vi "最終版.vi"() -> ()   [LabVIEW 2014]
uses:
  cloud.ctl
  heart.ctl
  <vilib>/Utility/inputDevices.llb/keyboardAcquire.vi
  <vilib>/Utility/inputDevices.llb/closeKeyboard.vi
panel:
  out "2-2":T1
  out "2-1":T2
  out "2":T1
  out "1":T2
  out "User 1":T3
  out "User 2":T3
  out "Ring 6":T4
  out "Ring 5":T5
  out "Ring 4":T5
  out "Ring 3":T4
  out "2jump":bool=TRUE
  out "User2 name":string
  out "User1 name":string
  out "人1生命":dbl
  out "人2生命":dbl
  out "heart 6":T6
  out "heart 5":T6
  out "heart 4":T6
  out "heart 3":T6
  out "heart 2":T6
  out "heart 1":T6
  out "雲  3":T7
  out "black hole":T8
  out "雲 2":T7
  out "雲":T7
  out "1jump":bool=TRUE
  out "火右飛 2":bool=TRUE
  out "火左飛 2":bool
  out "火左飛":bool
  out "火右飛":bool=TRUE
  in  "stop jump2":bool
  in  "stop jump1":bool
  in  "right/left 2":bool
  in  "人2":bool
  in  "right/left":bool
  in  "人1":bool
  in  "整個遊戲中止":bool
  # "587"
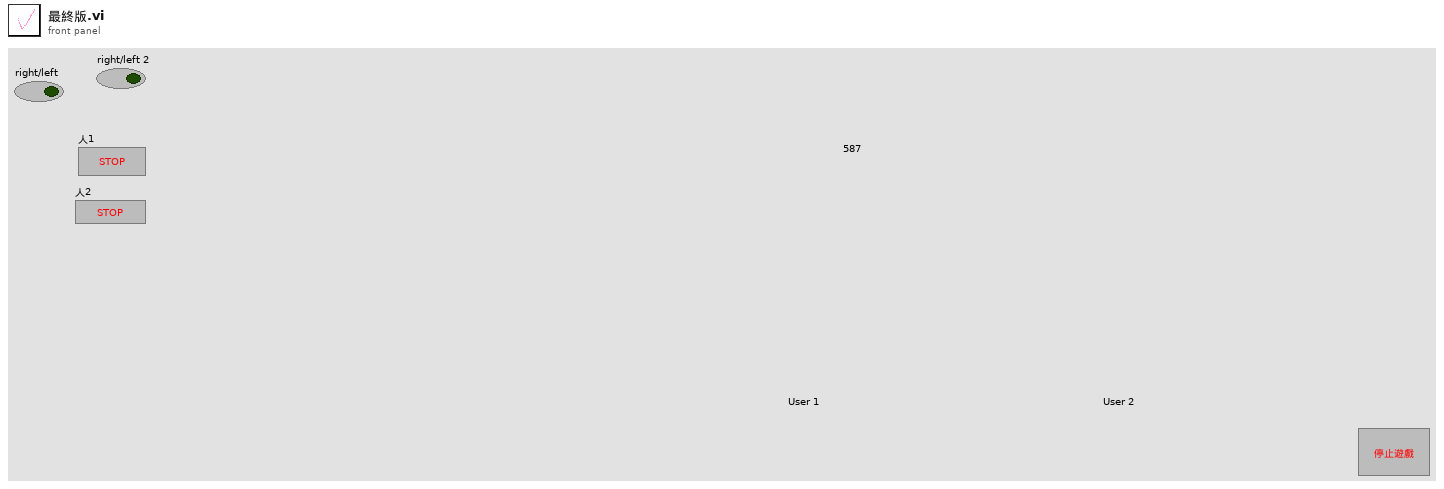
[diagram p1: front panel]
types:
  T1 = typedef "火焰2.ctl" = u16
  T2 = typedef "火焰.ctl" = u16
  T3 = typedef "Control 3.ctl" = u16
  T4 = typedef "窄短cloud.ctl" = u16
  T5 = typedef "窄cloud.ctl" = u16
  T6 = typedef "heart.ctl" = u16
  T7 = typedef "cloud.ctl" = u16
  T8 = typedef "Control 4.ctl" = u16
  T9 = enum16{"0", "1", "2", "3", "4", "5", "6", "7", "8", "9", "A", "B", "C", "D", "E", "F", "G", "H", "I", "J", "K", "L", "M", "N", "O", "P", "Q", "R", "S", "T", "U", "V", "W", "X", "Y", "Z", "F1", "F2", "F3", "F4", "F5", "F6", "F7", "F8", "F9", "F10", "F11", "F12", "F13", "F14", "F15", "ADD", "BACK", "BACKSLASH", "CAPITAL", "COMMA", "DECIMAL", "DELETE", "DIVIDE", "DOWN", "END", "EQUALS", "ESCAPE", "GRAVE (`)", "HOME", "INSERT", "LBRACKET", "LCONTROL", "LEFT", "L ALT", "LSHIFT", "LWIN", "MINUS", "MULTIPLY", "NEXT", "NUMLOCK", "NUMPAD_0", "NUMPAD_1", "NUMPAD_2", "NUMPAD_3", "NUMPAD_4", "NUMPAD_5", "NUMPAD_6", "NUMPAD_7", "NUMPAD_8", "NUMPAD_9", "PAUSE", "PERIOD", "PRIOR (PG UP)", "RBRACKET", "RCONTROL", "RETURN", "RIGHT", "R ALT", "RSHIFT", "RWIN", "SCROLL", "SEMICOLON", "SLASH", "SPACE", "SUBTRACT", "TAB", "UP", "ENTER (num pad)", "' (quote)"}
  T10 = enum16{"0", "1", "2", "3", "4", "5", "6", "7", "8", "9", "A", "B", "C", "D", "E", "F", "G", "H", "I", "J", "K", "L", "M", "N", "O", "P", "Q", "R", "S", "T", "U", "V", "W", "X", "Y", "Z", "F1", "F2", "F3", "F4", "F5", "F6", "F7", "F8", "F9", "F10", "F11", "F12", "F13", "F14", "F15", "ADD", "BACK", "BACKSLASH", "CAPITAL", "COMMA", "DECIMAL", "DELETE", "DIVIDE", "DOWN", "END", "EQUALS", "ESCAPE", "GRAVE (`)", "HOME", "INSERT", "LBRACKET", "LCONTROL", "LEFT", "L ALT", "LSHIFT", "LWIN", "MINUS", "MULTIPLY", "NEXT", "NUMLOCK", "NUMPAD_0", "NUMPAD_1", "NUMPAD_2", "NUMPAD_3", "NUMPAD_4", "NUMPAD_5", "NUMPAD_6", "NUMPAD_7", "NUMPAD_8", "NUMPAD_9", "PAUSE", "PERIOD", "PRIOR (PG UP)", "RBRACKET", "RCONTROL", "RETURN", "RIGHT", "R ALT", "RSHIFT", "RWIN", "SCROLL", "SEMICOLON", "SLASH", "SPACE", "SUBTRACT", "TAB", "UP", "ENTER (num pad)", "' (quote)"}[]
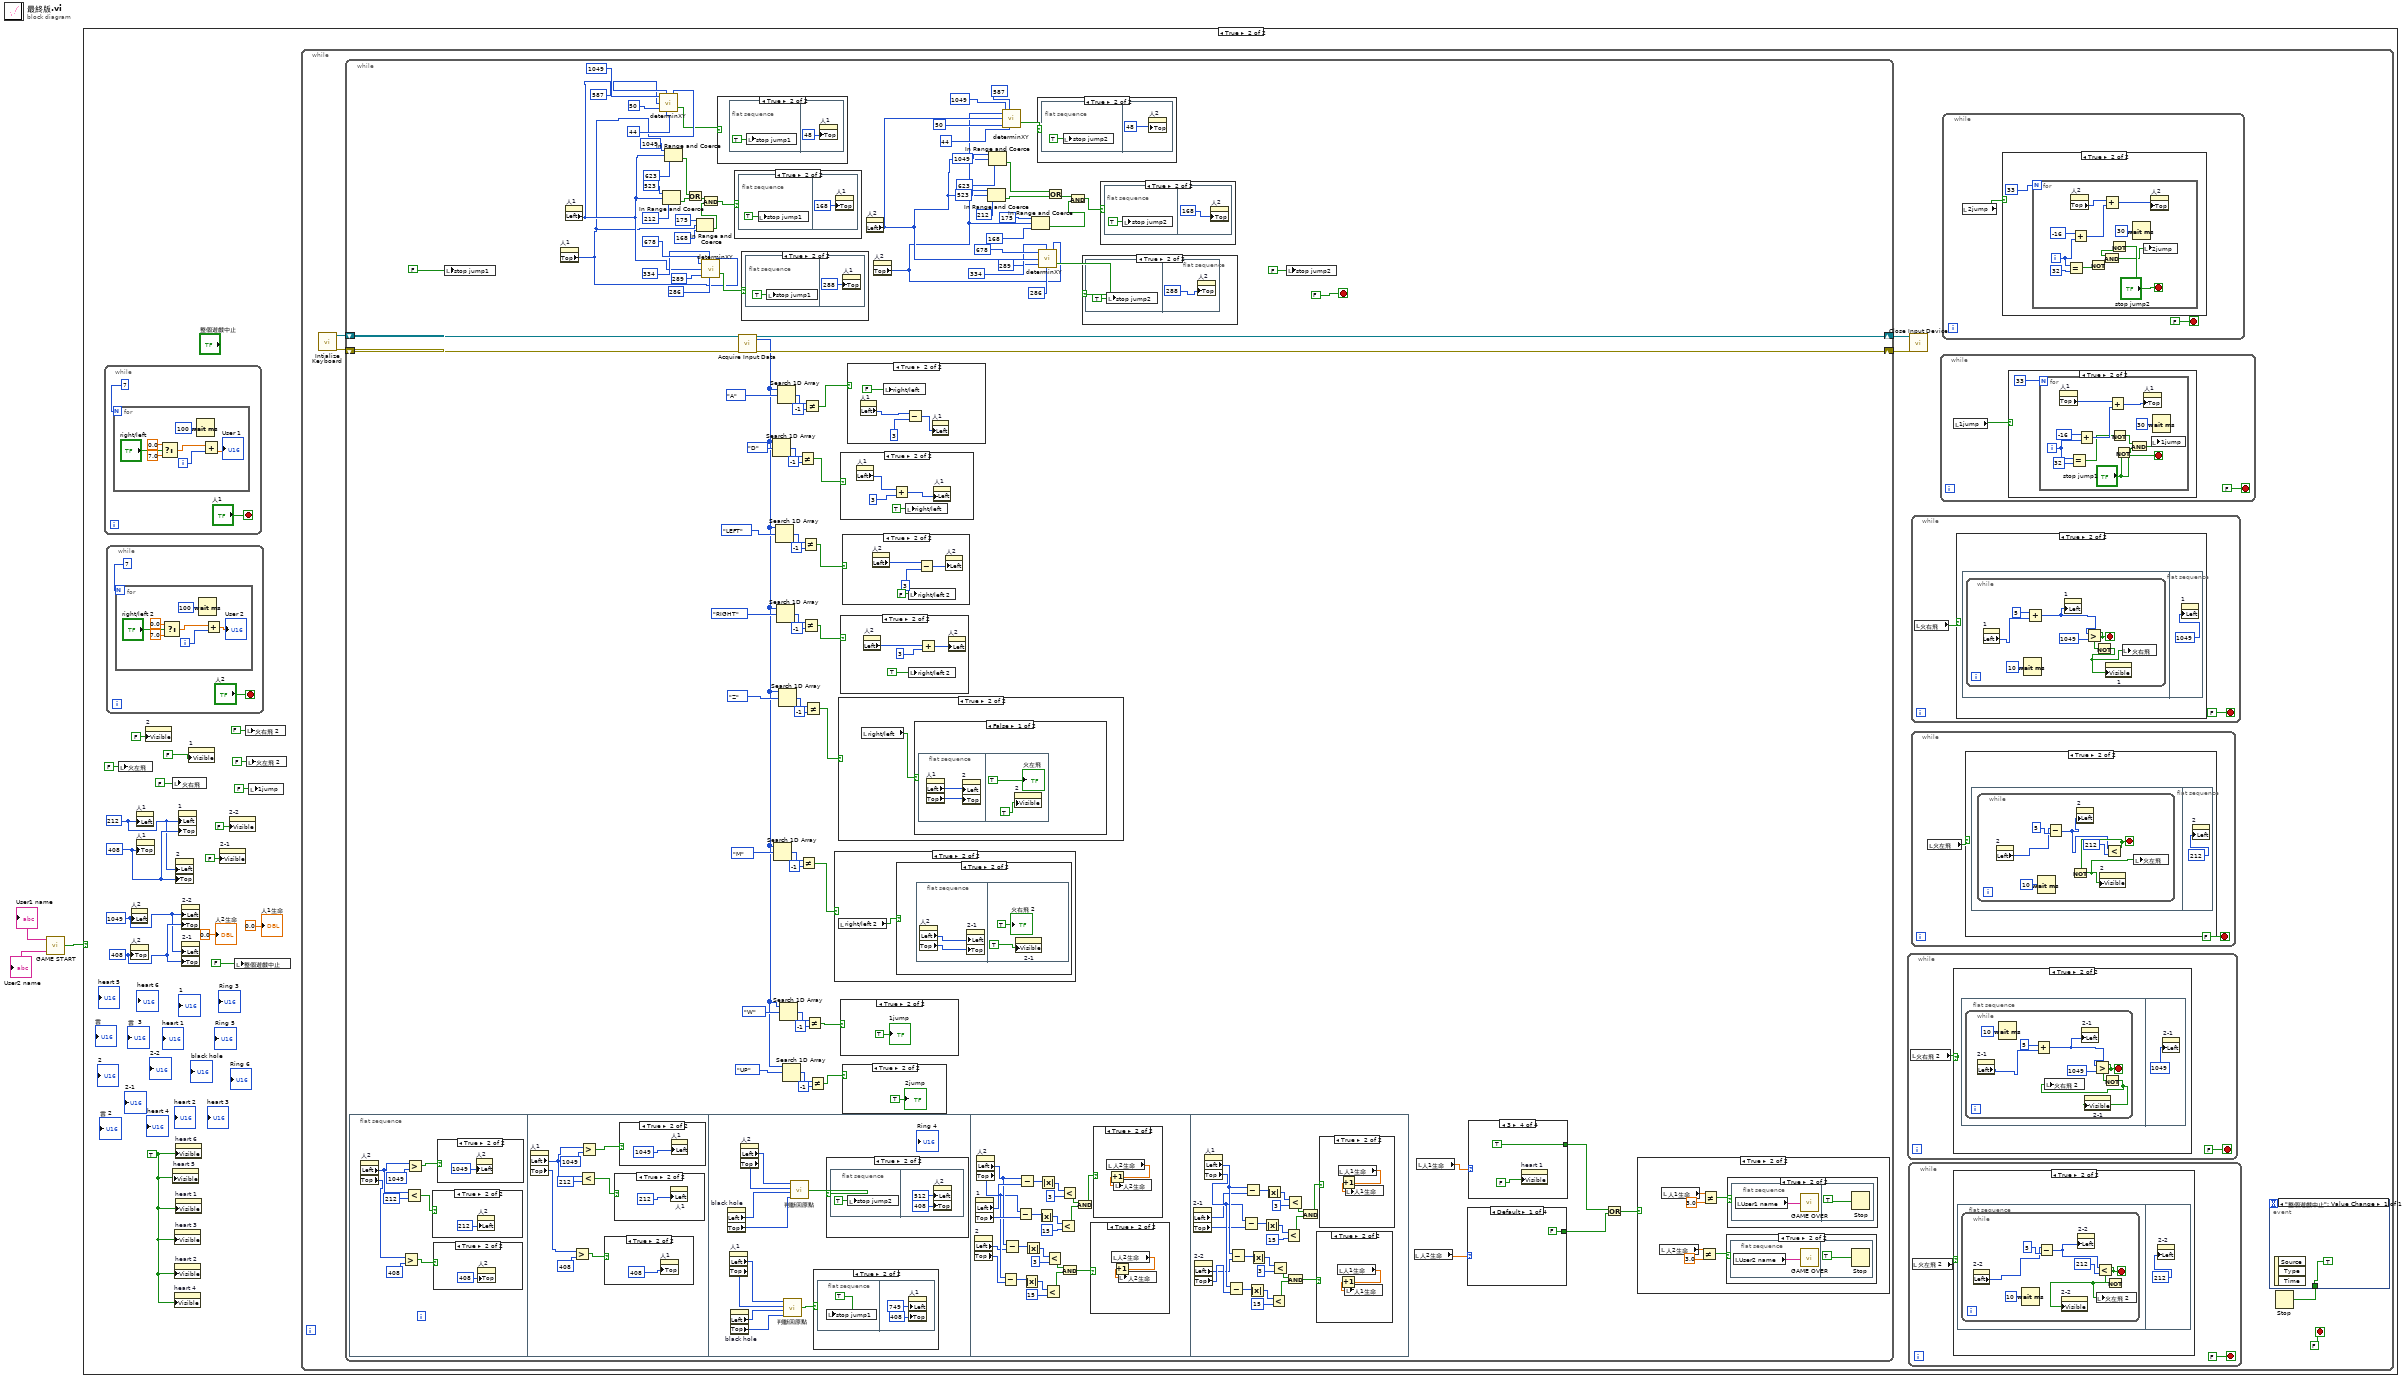
[diagram p0: block diagram]
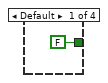
[diagram p13: hidden frame]
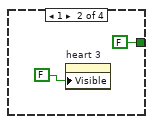
[diagram p14: hidden frame]
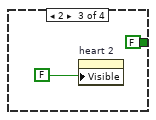
[diagram p15: hidden frame]
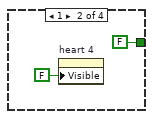
[diagram p16: hidden frame]
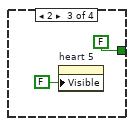
[diagram p17: hidden frame]
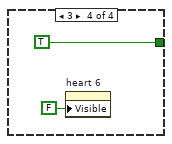
[diagram p18: hidden frame]
diagram:
  n1 = call "GAME START.vi"() -> ("stop 2"=w3:bool, "User2 name 2"=→"User2 name":string, "User1 name 2"=→"User1 name":string)  [unwired: 1 in]
  n2 = case shown="True" w3 {
    frame False {
    }
    frame True {
      w4 = TRUE ("Visible")
      w15 = 408 ("Position:Top")
      w14 = 1049 ("Position:Left")
      w13 = 408 ("Position:Top")
      w12 = 212 ("Position:Left")
      n3 = while {
        stop <- "人1" stop-if-true
        n4 = for {
          N: 7 -> [_]
          i -> [w28]
          n5 = Select(t=0.0, s="right/left", f=7.0) -> (s? t:f=w25:dbl)
          n6 = Wait (ms)(milliseconds to wait=u32 100) -> ()  [unwired: 1 out]
          n7 = Add(x=w25, y=w28) -> (x+y=→"User 1":dbl)
        }
      }
      n8 = while {
        stop <- "人2" stop-if-true
        n9 = for {
          N: 7 -> [_]
          i -> [w37]
          n10 = Select(t=0.0, s="right/left 2", f=7.0) -> (s? t:f=w35:dbl)
          n11 = Wait (ms)(milliseconds to wait=u32 100) -> ()  [unwired: 1 out]
          n12 = Add(x=w35, y=w37) -> (x+y=→"User 2":dbl)
        }
      }
      n13 = local write "火左飛"(FALSE ("火左飛")) -> ()
      n14 = property on="人2" class="Ring (strict)"("Top"=w15) -> ()  [unwired: 2 in, 2 out]
      n15 = property on="人2" class="Ring (strict)"("Left"=w14) -> ()  [unwired: 2 in, 2 out]
      n16 = property on="人1" class="Ring (strict)"("Left"=w12) -> ()  [unwired: 2 in, 2 out]
      n17 = property on="人1" class="Ring (strict)"("Top"=w13) -> ()  [unwired: 2 in, 2 out]
      n18 = property on="2" class="Ring (strict)"("Visible"=FALSE) -> ()  [unwired: 2 in, 2 out]
      n19 = local write "火右飛"(FALSE ("Boolean")) -> ()
      n20 = property on="heart 5" class="Ring (strict)"("Visible"=w4) -> ()  [unwired: 2 in, 2 out]
      n21 = property on="heart 4" class="Ring (strict)"("Visible"=w4) -> ()  [unwired: 2 in, 2 out]
      n22 = property on="heart 3" class="Ring (strict)"("Visible"=w4) -> ()  [unwired: 2 in, 2 out]
      n23 = property on="heart 2" class="Ring (strict)"("Visible"=w4) -> ()  [unwired: 2 in, 2 out]
      n24 = property on="heart 6" class="Ring (strict)"("Visible"=w4) -> ()  [unwired: 2 in, 2 out]
      n25 = property on="heart 1" class="Ring (strict)"("Visible"=w4) -> ()  [unwired: 2 in, 2 out]
      n26 = property on="2" class="Ring (strict)"("Left"=w12, "Top"=w13) -> ()  [unwired: 2 in, 2 out]
      n27 = property on="1" class="Ring (strict)"("Left"=w12, "Top"=w13) -> ()  [unwired: 2 in, 2 out]
      n28 = property on="2-2" class="Ring (strict)"("Left"=w14, "Top"=w15) -> ()  [unwired: 2 in, 2 out]
      n29 = property on="2-1" class="Ring (strict)"("Left"=w14, "Top"=w15) -> ()  [unwired: 2 in, 2 out]
      n30 = property on="1" class="Ring (strict)"("Visible"=FALSE) -> ()  [unwired: 2 in, 2 out]
      n31 = property on="2-1" class="Ring (strict)"("Visible"=FALSE) -> ()  [unwired: 2 in, 2 out]
      n32 = property on="2-2" class="Ring (strict)"("Visible"=FALSE) -> ()  [unwired: 2 in, 2 out]
      n33 = local write "整個遊戲中止"(FALSE ("整個遊戲中止")) -> ()
      n34 = local write "火右飛 2"(FALSE ("火右飛 2")) -> ()
      n35 = local write "火左飛 2"(FALSE ("火左飛 2")) -> ()
      n36 = local write "1jump"(FALSE ("1jump")) -> ()
      n37 = while {
        stop <- FALSE stop-if-true
        n38 = call <vilib>:"Intialize Keyboard.vi"() -> ("error out"=w43:errorcluster, "device ID"=w44:refnum<k1>)  [unwired: 10 in]
        n39 = while {
          shift-right: [w206] -> w41
          shift-left: w44 -> [w203]
          shift-right: [w205] -> w42
          shift-left: w43 -> [w204]
          stop <- FALSE stop-if-true
          n40 = flat-sequence {
            frame #0 {
              n41 = property on="人2" class="Ring (strict)"() -> ("Left"=w238:i32, "Top"=w233:i32)  [unwired: 2 in, 2 out]
              n42 = Greater?(x=w233, y=408) -> (0:w232:bool)
              n43 = Less?(x=w238, y=212) -> (x < y?=w235:bool)
              n44 = Greater?(x=w238, y=1049) -> (0:w236:bool)
              n45 = case shown="True" w235 {
                frame False {
                }
                frame True {
                  n46 = property on="人2" class="Ring (strict)"("Left"=212 ("Position:Left")) -> ()  [unwired: 2 in, 2 out]
                }
              }
              n47 = case shown="True" w232 {
                frame False {
                }
                frame True {
                  n48 = property on="人2" class="Ring (strict)"("Top"=408 ("Position:Left")) -> ()  [unwired: 2 in, 2 out]
                }
              }
              n49 = case shown="True" w236 {
                frame False {
                }
                frame True {
                  n50 = property on="人2" class="Ring (strict)"("Left"=1049 ("Position:Left")) -> ()  [unwired: 2 in, 2 out]
                }
              }
            }
            frame #1 {
              n51 = property on="人1" class="Ring (strict)"() -> ("Left"=w250:i32, "Top"=w243:i32)  [unwired: 2 in, 2 out]
              n52 = Greater?(x=w243, y=408) -> (0:w245:bool)
              n53 = Less?(x=w250, y=212) -> (x < y?=w249:bool)
              n54 = Greater?(x=w250, y=1049) -> (0:w248:bool)
              n55 = case shown="True" w245 {
                frame False {
                }
                frame True {
                  n56 = property on="人1" class="Ring (strict)"("Top"=408 ("Position:Left")) -> ()  [unwired: 2 in, 2 out]
                }
              }
              n57 = case shown="True" w249 {
                frame False {
                }
                frame True {
                  n58 = property on="人1" class="Ring (strict)"("Left"=212 ("Position:Left")) -> ()  [unwired: 2 in, 2 out]
                }
              }
              n59 = case shown="True" w248 {
                frame False {
                }
                frame True {
                  n60 = property on="人1" class="Ring (strict)"("Left"=1049 ("Position:Left")) -> ()  [unwired: 2 in, 2 out]
                }
              }
            }
            frame #2 {
              n61 = property on="black hole" class="Ring (strict)"() -> ("Left"=w261:i32, "Top"=w260:i32)  [unwired: 2 in, 2 out]
              n62 = property on="人1" class="Ring (strict)"() -> ("Left"=w254:i32, "Top"=w255:i32)  [unwired: 2 in, 2 out]
              n63 = property on="black hole" class="Ring (strict)"() -> ("Left"=w256:i32, "Top"=w257:i32)  [unwired: 2 in, 2 out]
              n64 = property on="人2" class="Ring (strict)"() -> ("Left"=w263:i32, "Top"=w262:i32)  [unwired: 2 in, 2 out]
              n65 = call "判斷回原點.vi"("¬}y"=w257, "¬}x"=w256, "人y"=w255, "人x"=w254) -> ("x .and. y?"=w258:bool)
              n66 = call "判斷回原點.vi"("¬}y"=w260, "¬}x"=w261, "人y"=w262, "人x"=w263) -> ("x .and. y?"=w259:bool)
              n67 = case shown="True" w258 {
                frame False {
                }
                frame True {
                  n68 = flat-sequence {
                    frame #0 {
                      n69 = local write "stop jump1"(TRUE) -> ()
                    }
                    frame #1 {
                      n70 = property on="人1" class="Ring (strict)"("Left"=749 ("Position:Left"), "Top"=408 ("Position:Top")) -> ()  [unwired: 2 in, 2 out]
                    }
                  }
                }
              }
              n71 = case shown="True" w259 {
                frame False {
                }
                frame True {
                  n72 = flat-sequence {
                    frame #0 {
                      n73 = local write "stop jump2"(TRUE ("stop jump2")) -> ()
                    }
                    frame #1 {
                      n74 = property on="人2" class="Ring (strict)"("Left"=512 ("Position:Left"), "Top"=408 ("Position:Top")) -> ()  [unwired: 2 in, 2 out]
                    }
                  }
                }
              }
            }
            frame #3 {
              n75 = property on="2" class="Ring (strict)"() -> ("Left"=w271:i32, "Top"=w270:i32)  [unwired: 2 in, 2 out]
              n76 = property on="1" class="Ring (strict)"() -> ("Left"=w293:i32, "Top"=w286:i32)  [unwired: 2 in, 2 out]
              n77 = property on="人2" class="Ring (strict)"() -> ("Left"=w273:i32, "Top"=w272:i32)  [unwired: 2 in, 2 out]
              n78 = Subtract(x=w272, y=w270) -> (x-y=w280:i32)
              n79 = Subtract(x=w273, y=w271) -> (x-y=w275:i32)
              n80 = Subtract(x=w272, y=w286) -> (x-y=w287:i32)
              n81 = Subtract(x=w273, y=w293) -> (x-y=w292:i32)
              n82 = Absolute Value(x=w280) -> (abs(x)=w279:i32)
              n83 = Absolute Value(x=w275) -> (abs(x)=w276:i32)
              n84 = Absolute Value(x=w287) -> (abs(x)=w288:i32)
              n85 = Absolute Value(x=w292) -> (abs(x)=w291:i32)
              n86 = Less?(x=w279, y=15) -> (x < y?=w282:bool)
              n87 = Less?(x=w276, y=3) -> (x < y?=w281:bool)
              n88 = Less?(x=w288, y=15) -> (x < y?=w284:bool)
              n89 = Less?(x=w291, y=3) -> (x < y?=w285:bool)
              n90 = And(x=w281, y=w282) -> (x .and. y?=w274:bool)
              n91 = And(x=w285, y=w284) -> (x .and. y?=w283:bool)
              n92 = case shown="True" w274 {
                frame False {
                }
                frame True {
                  n93 = local read "人2生命"() -> (w295:dbl)
                  n94 = Increment(x=w295) -> (x+1=w294:dbl)
                  n95 = local write "人2生命"(w294) -> ()
                }
              }
              n96 = case shown="True" w283 {
                frame False {
                }
                frame True {
                  n97 = local read "人2生命"() -> (w296:dbl)
                  n98 = Increment(x=w296) -> (x+1=w297:dbl)
                  n99 = local write "人2生命"(w297) -> ()
                }
              }
            }
            frame #4 {
              n100 = property on="2-1" class="Ring (strict)"() -> ("Left"=w300:i32, "Top"=w301:i32)  [unwired: 2 in, 2 out]
              n101 = property on="2-2" class="Ring (strict)"() -> ("Left"=w298:i32, "Top"=w299:i32)  [unwired: 2 in, 2 out]
              n102 = property on="人1" class="Ring (strict)"() -> ("Left"=w303:i32, "Top"=w302:i32)  [unwired: 2 in, 2 out]
              n103 = Subtract(x=w302, y=w299) -> (x-y=w315:i32)
              n104 = Subtract(x=w303, y=w298) -> (x-y=w320:i32)
              n105 = Subtract(x=w302, y=w301) -> (x-y=w309:i32)
              n106 = Subtract(x=w303, y=w300) -> (x-y=w304:i32)
              n107 = Absolute Value(x=w315) -> (abs(x)=w316:i32)
              n108 = Absolute Value(x=w320) -> (abs(x)=w319:i32)
              n109 = Absolute Value(x=w309) -> (abs(x)=w308:i32)
              n110 = Absolute Value(x=w304) -> (abs(x)=w305:i32)
              n111 = Less?(x=w316, y=15) -> (x < y?=w313:bool)
              n112 = Less?(x=w319, y=3) -> (x < y?=w314:bool)
              n113 = Less?(x=w308, y=15) -> (x < y?=w311:bool)
              n114 = Less?(x=w305, y=3) -> (x < y?=w310:bool)
              n115 = And(x=w314, y=w313) -> (x .and. y?=w321:bool)
              n116 = And(x=w310, y=w311) -> (x .and. y?=w312:bool)
              n117 = case shown="True" w321 {
                frame False {
                }
                frame True {
                  n118 = local read "人1生命"() -> (w323:dbl)
                  n119 = Increment(x=w323) -> (x+1=w322:dbl)
                  n120 = local write "人1生命"(w322) -> ()
                }
              }
              n121 = case shown="True" w312 {
                frame False {
                }
                frame True {
                  n122 = local read "人1生命"() -> (w324:dbl)
                  n123 = Increment(x=w324) -> (x+1=w325:dbl)
                  n124 = local write "人1生命"(w325) -> ()
                }
              }
            }
          }
          n125 = local write "stop jump1"(FALSE ("stop jump1")) -> ()
          n126 = property on="人1" class="Ring (strict)"() -> ("Top"=w139:i32)  [unwired: 2 in, 2 out]
          n127 = property on="人1" class="Ring (strict)"() -> ("Left"=w142:i32)  [unwired: 2 in, 2 out]
          n128 = call "determinXY.vi"("x max"=1049 ("upper limit"), "x min"=587 ("lower limit"), "x"=w142, "y max"=50 ("upper limit"), "y min"=44 ("lower limit"), "y"=w139) -> ("result"=w138:bool)
          n129 = In Range and Coerce(upper limit=523, x=w142, lower limit=212) -> (In Range?=w177:bool)  [unwired: 1 out]
          n130 = In Range and Coerce(upper limit=1049, x=w142, lower limit=623) -> (In Range?=w178:bool)  [unwired: 1 out]
          n131 = Or(x=w178, y=w177) -> (x .or. y?=w179:bool)
          n132 = In Range and Coerce(upper limit=175, x=w139, lower limit=168 ("y")) -> (In Range?=w183:bool)  [unwired: 1 out]
          n133 = And(x=w179, y=w183) -> (x .and. y?=w176:bool)
          n134 = call "determinXY.vi"("x max"=678 ("upper limit"), "x min"=334 ("lower limit"), "x"=w142, "y max"=289 ("upper limit"), "y min"=286 ("y"), "y"=w139) -> ("result"=w145:bool)
          n135 = case shown="True" w138 {
            frame False {
            }
            frame True {
              n136 = flat-sequence {
                frame #0 {
                  n137 = local write "stop jump1"(TRUE ("stop jump1")) -> ()
                }
                frame #1 {
                  n138 = property on="人1" class="Ring (strict)"("Top"=48 ("Position:Top")) -> ()  [unwired: 2 in, 2 out]
                }
              }
            }
          }
          n139 = case shown="True" w176 {
            frame False {
            }
            frame True {
              n140 = flat-sequence {
                frame #0 {
                  n141 = local write "stop jump1"(TRUE ("stop jump1")) -> ()
                }
                frame #1 {
                  n142 = property on="人1" class="Ring (strict)"("Top"=168 ("Position:Top")) -> ()  [unwired: 2 in, 2 out]
                }
              }
            }
          }
          n143 = call-poly <vilib>:"Acquire Input Data.vi"("device ID"=w203, "error in (no error)"=w204) -> ("device ID"=w206:refnum<k1>, "keys pressed"=w119:T10, "error out"=w205:errorcluster)  [unwired: 15 in]
          n144 = case shown="True" w145 {
            frame False {
            }
            frame True {
              n145 = flat-sequence {
                frame #0 {
                  n146 = local write "stop jump1"(TRUE ("stop jump1")) -> ()
                }
                frame #1 {
                  n147 = property on="人1" class="Ring (strict)"("Top"=288 ("Position:Top")) -> ()  [unwired: 2 in, 2 out]
                }
              }
            }
          }
          n148 = Search 1D Array(1D array=w119, element=T9."D") -> (index of element=w197:i32)  [unwired: 1 in]
          n149 = Search 1D Array(1D array=w119, element=T9."M") -> (index of element=w159:i32)  [unwired: 1 in]
          n150 = Search 1D Array(1D array=w119, element=T9."LEFT") -> (index of element=w194:i32)  [unwired: 1 in]
          n151 = Search 1D Array(1D array=w119, element=T9."RIGHT") -> (index of element=w190:i32)  [unwired: 1 in]
          n152 = Search 1D Array(1D array=w119, element=T9."A") -> (index of element=w200:i32)  [unwired: 1 in]
          n153 = Search 1D Array(1D array=w119, element=T9."Z") -> (index of element=w162:i32)  [unwired: 1 in]
          n154 = Search 1D Array(1D array=w119, element=T9."W") -> (index of element=w152:i32)  [unwired: 1 in]
          n155 = Search 1D Array(1D array=w119, element=T9."UP") -> (index of element=w121:i32)  [unwired: 1 in]
          n156 = Not Equal?(x=w197, y=-1) -> (x != y?=w155:bool)
          n157 = Not Equal?(x=w159, y=-1) -> (x != y?=w157:bool)
          n158 = Not Equal?(x=w194, y=-1) -> (x != y?=w192:bool)
          n159 = Not Equal?(x=w190, y=-1) -> (x != y?=w188:bool)
          n160 = Not Equal?(x=w200, y=-1) -> (x != y?=w156:bool)
          n161 = Not Equal?(x=w162, y=-1) -> (x != y?=w154:bool)
          n162 = Not Equal?(x=w152, y=-1) -> (x != y?=w150:bool)
          n163 = Not Equal?(x=w121, y=-1) -> (x != y?=w118:bool)
          n164 = case shown="True" w157 {
            frame False {
            }
            frame True {
              n165 = local read "right/left 2"() -> (w327:bool)
              n166 = case shown="True" w327 {
                frame False {
                  n167 = flat-sequence {
                    frame #0 {
                      n168 = property on="人2" class="Ring (strict)"() -> ("Left"=w329:i32, "Top"=w328:i32)  [unwired: 2 in, 2 out]
                      n169 = property on="2-2" class="Ring (strict)"("Left"=w329, "Top"=w328) -> ()  [unwired: 2 in, 2 out]
                    }
                    frame #1 {
                      n170 = property on="2-2" class="Ring (strict)"("Visible"=TRUE) -> ()  [unwired: 2 in, 2 out]
                      "火左飛 2" <- TRUE
                    }
                  }
                }
                frame True {
                  n171 = flat-sequence {
                    frame #0 {
                      n172 = property on="人2" class="Ring (strict)"() -> ("Left"=w333:i32, "Top"=w332:i32)  [unwired: 2 in, 2 out]
                      n173 = property on="2-1" class="Ring (strict)"("Left"=w333, "Top"=w332) -> ()  [unwired: 2 in, 2 out]
                    }
                    frame #1 {
                      n174 = property on="2-1" class="Ring (strict)"("Visible"=TRUE) -> ()  [unwired: 2 in, 2 out]
                      "火右飛 2" <- TRUE
                    }
                  }
                }
              }
            }
          }
          n175 = case shown="True" w154 {
            frame False {
            }
            frame True {
              n176 = local read "right/left"() -> (w336:bool)
              n177 = case shown="False" w336 {
                frame False {
                  n178 = flat-sequence {
                    frame #0 {
                      n179 = property on="人1" class="Ring (strict)"() -> ("Left"=w338:i32, "Top"=w337:i32)  [unwired: 2 in, 2 out]
                      n180 = property on="2" class="Ring (strict)"("Left"=w338, "Top"=w337) -> ()  [unwired: 2 in, 2 out]
                    }
                    frame #1 {
                      n181 = property on="2" class="Ring (strict)"("Visible"=TRUE) -> ()  [unwired: 2 in, 2 out]
                      "火左飛" <- TRUE
                    }
                  }
                }
                frame True {
                  n182 = flat-sequence {
                    frame #0 {
                      n183 = property on="人1" class="Ring (strict)"() -> ("Left"=w342:i32, "Top"=w341:i32)  [unwired: 2 in, 2 out]
                      n184 = property on="1" class="Ring (strict)"("Left"=w342, "Top"=w341) -> ()  [unwired: 2 in, 2 out]
                    }
                    frame #1 {
                      n185 = property on="1" class="Ring (strict)"("Visible"=TRUE) -> ()  [unwired: 2 in, 2 out]
                      "火右飛" <- TRUE
                    }
                  }
                }
              }
            }
          }
          n186 = case shown="True" w150 {
            frame False {
            }
            frame True {
              "1jump" <- TRUE
            }
          }
          n187 = case shown="True" w155 {
            frame False {
            }
            frame True {
              n188 = property on="人1" class="Ring (strict)"() -> ("Left"=w367:i32)  [unwired: 2 in, 2 out]
              n189 = Add(x=w367, y=3) -> (x+y=w366:i32)
              n190 = local write "right/left"(TRUE ("right/left")) -> ()
              n191 = property on="人1" class="Ring (strict)"("Left"=w366) -> ()  [unwired: 2 in, 2 out]
            }
          }
          n192 = case shown="True" w188 {
            frame False {
            }
            frame True {
              n193 = property on="人2" class="Ring (strict)"() -> ("Left"=w359:i32)  [unwired: 2 in, 2 out]
              n194 = local write "right/left 2"(TRUE ("人1 right 2")) -> ()
              n195 = Add(x=w359, y=3) -> (x+y=w358:i32)
              n196 = property on="人2" class="Ring (strict)"("Left"=w358) -> ()  [unwired: 2 in, 2 out]
            }
          }
          n197 = case shown="True" w192 {
            frame False {
            }
            frame True {
              n198 = property on="人2" class="Ring (strict)"() -> ("Left"=w363:i32)  [unwired: 2 in, 2 out]
              n199 = local write "right/left 2"(FALSE ("right/left")) -> ()
              n200 = Subtract(x=w363, y=3) -> (x-y=w362:i32)
              n201 = property on="人2" class="Ring (strict)"("Left"=w362) -> ()  [unwired: 2 in, 2 out]
            }
          }
          n202 = case shown="True" w118 {
            frame False {
            }
            frame True {
              "2jump" <- TRUE ("2jump")
            }
          }
          n203 = case shown="True" w156 {
            frame False {
            }
            frame True {
              n204 = property on="人1" class="Ring (strict)"() -> ("Left"=w370:i32)  [unwired: 2 in, 2 out]
              n205 = local write "right/left"(FALSE ("人1 right 2")) -> ()
              n206 = Subtract(x=w370, y=3) -> (x-y=w369:i32)
              n207 = property on="人1" class="Ring (strict)"("Left"=w369) -> ()  [unwired: 2 in, 2 out]
            }
          }
          n208 = property on="人2" class="Ring (strict)"() -> ("Left"=w132:i32)  [unwired: 2 in, 2 out]
          n209 = property on="人2" class="Ring (strict)"() -> ("Top"=w117:i32)  [unwired: 2 in, 2 out]
          n210 = In Range and Coerce(upper limit=523, x=w132, lower limit=212) -> (In Range?=w166:bool)  [unwired: 1 out]
          n211 = In Range and Coerce(upper limit=1049, x=w132, lower limit=623) -> (In Range?=w167:bool)  [unwired: 1 out]
          n212 = call "determinXY.vi"("x max"=1049 ("upper limit"), "x min"=587 ("lower limit"), "x"=w132, "y max"=50 ("upper limit"), "y min"=44 ("lower limit"), "y"=w117) -> ("result"=w134:bool)
          n213 = In Range and Coerce(upper limit=175, x=w117, lower limit=168 ("y")) -> (In Range?=w171:bool)  [unwired: 1 out]
          n214 = case shown="True" w134 {
            frame False {
            }
            frame True {
              n215 = flat-sequence {
                frame #0 {
                  n216 = local write "stop jump2"(TRUE ("stop jump1")) -> ()
                }
                frame #1 {
                  n217 = property on="人2" class="Ring (strict)"("Top"=48 ("Position:Top")) -> ()  [unwired: 2 in, 2 out]
                }
              }
            }
          }
          n218 = call "determinXY.vi"("x max"=678 ("upper limit"), "x min"=334 ("lower limit"), "x"=w132, "y max"=289 ("upper limit"), "y min"=286 ("y"), "y"=w117) -> ("result"=w128:bool)
          n219 = Or(x=w167, y=w166) -> (x .or. y?=w168:bool)
          n220 = And(x=w168, y=w171) -> (x .and. y?=w165:bool)
          n221 = case shown="True" w128 {
            frame False {
            }
            frame True {
              n222 = flat-sequence {
                frame #0 {
                  n223 = local write "stop jump2"(TRUE ("stop jump1")) -> ()
                }
                frame #1 {
                  n224 = property on="人2" class="Ring (strict)"("Top"=288 ("Position:Top")) -> ()  [unwired: 2 in, 2 out]
                }
              }
            }
          }
          n225 = case shown="True" w165 {
            frame False {
            }
            frame True {
              n226 = flat-sequence {
                frame #0 {
                  n227 = local write "stop jump2"(TRUE ("stop jump1")) -> ()
                }
                frame #1 {
                  n228 = property on="人2" class="Ring (strict)"("Top"=168 ("Position:Top")) -> ()  [unwired: 2 in, 2 out]
                }
              }
            }
          }
          n229 = local write "stop jump2"(FALSE ("stop jump1 2")) -> ()
          n230 = local read "人2生命"() -> (w127:dbl)
          n231 = local read "人1生命"() -> (w126:dbl)
          n232 = case shown="Default" w127 {
            tunnel: [FALSE ("整個遊戲中止") FALSE ("整個遊戲中止") FALSE ("整個遊戲中止") TRUE ("整個遊戲中止")] -> w124
            frame Default {
            }
            frame 1 {
              n233 = property on="heart 4" class="Ring (strict)"("Visible"=FALSE) -> ()  [unwired: 2 in, 2 out]
            }
            frame 2 {
              n234 = property on="heart 5" class="Ring (strict)"("Visible"=FALSE) -> ()  [unwired: 2 in, 2 out]
            }
            frame 3 {
              n235 = property on="heart 6" class="Ring (strict)"("Visible"=FALSE) -> ()  [unwired: 2 in, 2 out]
            }
          }
          n236 = case shown="3" w126 {
            tunnel: [FALSE ("整個遊戲中止") FALSE ("整個遊戲中止") FALSE ("整個遊戲中止") TRUE ("整個遊戲中止")] -> w125
            frame Default {
            }
            frame 1 {
              n237 = property on="heart 3" class="Ring (strict)"("Visible"=FALSE) -> ()  [unwired: 2 in, 2 out]
            }
            frame 2 {
              n238 = property on="heart 2" class="Ring (strict)"("Visible"=FALSE) -> ()  [unwired: 2 in, 2 out]
            }
            frame 3 {
              n239 = property on="heart 1" class="Ring (strict)"("Visible"=FALSE) -> ()  [unwired: 2 in, 2 out]
            }
          }
          n240 = Or(x=w125, y=w124) -> (x .or. y?=w123:bool)
          n241 = case shown="True" w123 {
            frame False {
            }
            frame True {
              n242 = local read "人2生命"() -> (w208:dbl)
              n243 = local read "人1生命"() -> (w213:dbl)
              n244 = Not Equal?(x=w208, y=3.0) -> (x != y?=w210:bool)
              n245 = Not Equal?(x=w213, y=3.0) -> (x != y?=w211:bool)
              n246 = case shown="True" w210 {
                frame False {
                }
                frame True {
                  n247 = flat-sequence {
                    frame #0 {
                      n248 = local read "User2 name"() -> (w214:string)
                      n249 = call "GAME OVER.vi"("name"=w214) -> ()  [unwired: 1 in]
                    }
                    frame #1 {
                      n250 = Stop(stop? (T)=TRUE) -> ()
                    }
                  }
                }
              }
              n251 = case shown="True" w211 {
                frame False {
                }
                frame True {
                  n252 = flat-sequence {
                    frame #0 {
                      n253 = local read "User1 name"() -> (w216:string)
                      n254 = call "GAME OVER.vi"("name"=w216) -> ()  [unwired: 1 in]
                    }
                    frame #1 {
                      n255 = Stop(stop? (T)=TRUE) -> ()
                    }
                  }
                }
              }
            }
          }
        }
        n256 = while {
          stop <- FALSE stop-if-true
          n257 = local read "火右飛 2"() -> (w72:bool)
          n258 = case shown="True" w72 {
            frame False {
            }
            frame True {
              n259 = flat-sequence {
                frame #0 {
                  n260 = while {
                    stop <- w77 stop-if-true
                    n261 = property on="2-1" class="Ring (strict)"() -> ("Left"=w76:i32)  [unwired: 2 in, 2 out]
                    n262 = Wait (ms)(milliseconds to wait=u32 10) -> ()  [unwired: 1 out]
                    n263 = Add(x=5, y=w76) -> (x+y=w75:i32)
                    n264 = property on="2-1" class="Ring (strict)"("Left"=w75) -> ()  [unwired: 2 in, 2 out]
                    n265 = Greater?(x=w75, y=1049) -> (0:w77:bool)
                    n266 = Not(x=w77) -> (.not. x?=w73:bool)
                    n267 = local write "火右飛 2"(w73) -> ()
                    n268 = property on="2-1" class="Ring (strict)"("Visible"=w73) -> ()  [unwired: 2 in, 2 out]
                  }
                }
                frame #1 {
                  n269 = property on="2-1" class="Ring (strict)"("Left"=1049 ("y")) -> ()  [unwired: 2 in, 2 out]
                }
              }
            }
          }
        }
        n270 = while {
          stop <- FALSE stop-if-true
          n271 = local read "火左飛 2"() -> (w62:bool)
          n272 = case shown="True" w62 {
            frame False {
            }
            frame True {
              n273 = flat-sequence {
                frame #0 {
                  n274 = while {
                    stop <- w69 stop-if-true
                    n275 = property on="2-2" class="Ring (strict)"() -> ("Left"=w67:i32)  [unwired: 2 in, 2 out]
                    n276 = Wait (ms)(milliseconds to wait=u32 10) -> ()  [unwired: 1 out]
                    n277 = Subtract(x=w67, y=5 ("x")) -> (x-y=w64:i32)
                    n278 = property on="2-2" class="Ring (strict)"("Left"=w64) -> ()  [unwired: 2 in, 2 out]
                    n279 = Less?(x=w64, y=212) -> (x < y?=w69:bool)
                    n280 = Not(x=w69) -> (.not. x?=w63:bool)
                    n281 = property on="2-2" class="Ring (strict)"("Visible"=w63) -> ()  [unwired: 2 in, 2 out]
                    n282 = local write "火左飛 2"(w63) -> ()
                  }
                }
                frame #1 {
                  n283 = property on="2-2" class="Ring (strict)"("Left"=212 ("y")) -> ()  [unwired: 2 in, 2 out]
                }
              }
            }
          }
        }
        n284 = call-poly <vilib>:"Close Input Device.vi"("error in (no error)"=w42, "device ID"=w41) -> ()  [unwired: 8 in, 1 out]
        n285 = while {
          stop <- FALSE stop-if-true
          n286 = local read "火右飛"() -> (w82:bool)
          n287 = case shown="True" w82 {
            frame False {
            }
            frame True {
              n288 = flat-sequence {
                frame #0 {
                  n289 = while {
                    stop <- w87 stop-if-true
                    n290 = property on="1" class="Ring (strict)"() -> ("Left"=w86:i32)  [unwired: 2 in, 2 out]
                    n291 = Wait (ms)(milliseconds to wait=u32 10) -> ()  [unwired: 1 out]
                    n292 = Add(x=5, y=w86) -> (x+y=w85:i32)
                    n293 = property on="1" class="Ring (strict)"("Left"=w85) -> ()  [unwired: 2 in, 2 out]
                    n294 = Greater?(x=w85, y=1049) -> (0:w87:bool)
                    n295 = Not(x=w87) -> (.not. x?=w83:bool)
                    n296 = property on="1" class="Ring (strict)"("Visible"=w83) -> ()  [unwired: 2 in, 2 out]
                    n297 = local write "火右飛"(w83) -> ()
                  }
                }
                frame #1 {
                  n298 = property on="1" class="Ring (strict)"("Left"=1049 ("y")) -> ()  [unwired: 2 in, 2 out]
                }
              }
            }
          }
        }
        n299 = while {
          stop <- FALSE stop-if-true
          n300 = local read "火左飛"() -> (w92:bool)
          n301 = case shown="True" w92 {
            frame False {
            }
            frame True {
              n302 = flat-sequence {
                frame #0 {
                  n303 = while {
                    stop <- w99 stop-if-true
                    n304 = property on="2" class="Ring (strict)"() -> ("Left"=w97:i32)  [unwired: 2 in, 2 out]
                    n305 = Wait (ms)(milliseconds to wait=u32 10) -> ()  [unwired: 1 out]
                    n306 = Subtract(x=w97, y=5 ("x")) -> (x-y=w94:i32)
                    n307 = property on="2" class="Ring (strict)"("Left"=w94) -> ()  [unwired: 2 in, 2 out]
                    n308 = Less?(x=w94, y=212) -> (x < y?=w99:bool)
                    n309 = Not(x=w99) -> (.not. x?=w93:bool)
                    n310 = property on="2" class="Ring (strict)"("Visible"=w93) -> ()  [unwired: 2 in, 2 out]
                    n311 = local write "火左飛"(w93) -> ()
                  }
                }
                frame #1 {
                  n312 = property on="2" class="Ring (strict)"("Left"=212 ("y")) -> ()  [unwired: 2 in, 2 out]
                }
              }
            }
          }
        }
        n313 = while {
          stop <- FALSE stop-if-true
          n314 = local read "1jump"() -> (w46:bool)
          n315 = case shown="True" w46 {
            frame False {
            }
            frame True {
              n316 = for {
                N: 33 -> [_]
                i -> [w54]
                stop <- "stop jump1" stop-if-true
                n317 = property on="人1" class="Ring (strict)"() -> ("Top"=w57:i32)  [unwired: 2 in, 2 out]
                n318 = Equal?(x=w54, y=32) -> (x = y?=w52:bool)
                n319 = Add(x=-16, y=w54) -> (x+y=w59:i32)
                n320 = Add(x=w57, y=w59) -> (x+y=w56:i32)
                n321 = Not(x=w52) -> (.not. x?=w51:bool)
                n322 = Not(x="stop jump1") -> (.not. x?=w50:bool)
                n323 = And(x=w51, y=w50) -> (x .and. y?=w49:bool)
                n324 = property on="人1" class="Ring (strict)"("Top"=w56) -> ()  [unwired: 2 in, 2 out]
                n325 = local write "1jump"(w49) -> ()
                n326 = Wait (ms)(milliseconds to wait=u32 30) -> ()  [unwired: 1 out]
              }
            }
          }
        }
        n327 = while {
          stop <- FALSE stop-if-true
          n328 = local read "2jump"() -> (w101:bool)
          n329 = case shown="True" w101 {
            frame False {
            }
            frame True {
              n330 = for {
                N: 33 -> [_]
                i -> [w109]
                stop <- "stop jump2" stop-if-true
                n331 = Equal?(x=w109, y=32) -> (x = y?=w108:bool)
                n332 = property on="人2" class="Ring (strict)"() -> ("Top"=w112:i32)  [unwired: 2 in, 2 out]
                n333 = Add(x=-16, y=w109) -> (x+y=w114:i32)
                n334 = Not(x=w108) -> (.not. x?=w107:bool)
                n335 = Add(x=w112, y=w114) -> (x+y=w111:i32)
                n336 = Not(x="stop jump2") -> (.not. x?=w106:bool)
                n337 = And(x=w106, y=w107) -> (x .and. y?=w104:bool)
                n338 = Wait (ms)(milliseconds to wait=u32 30) -> ()  [unwired: 1 out]
                n339 = local write "2jump"(w104) -> ()
                n340 = property on="人2" class="Ring (strict)"("Top"=w111) -> ()  [unwired: 2 in, 2 out]
              }
            }
          }
        }
        n341 = event shown="[0] \"整個遊戲中止\": Value Change" {
          selector: _ -> [_]
          dyn-events: _ -> [_]
          timeout: _ -> [_]
          tunnel: [TRUE] -> w40
          event "整個遊戲中止": Value Change {
            n342 = event-data() -> ()  [unwired: 1 in, 3 out]
          }
        }
        n343 = Stop(stop? (T)=w40) -> ()
      }
      "人2生命" <- 0.0 ("人1生命")
      "人1生命" <- 0.0 ("人2生命")
    }
  }
